vi "Set VLIM.vi"(8 "error in":errorcluster, 10 "VLIM":sgl, 11 "SR 3XX HVPS in":refnum<class "SR 3XX HVPS.lvclass">) -> (0 "error out":errorcluster, 3 "SR 3XX HVPS out":refnum<class "SR 3XX HVPS.lvclass">)   [LabVIEW 2014, in "SR 3XX HVPS.lvclass"]
doc: "The VLIM command sets the value of the voltage limit to x where x is the value in Volts. The sign of value x MUST match the PS300’s polarity setting.As with front panel control, the VLIM value must be greater than or equal to the VSET value or an execution error will be returned."
uses:
  SR 3XX HVPS.lvclass
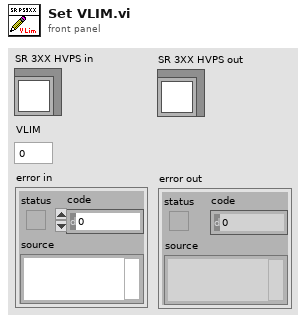
[diagram p1: front panel]
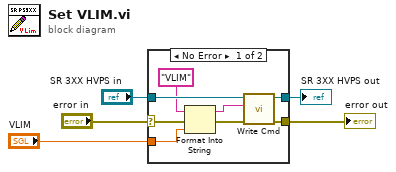
[diagram p0: block diagram]
diagram:
  n1 = case shown="No Error" "error in" {
    selector: "error in" -> [w7 w15]
    tunnel: [w11 w15] -> w4
    tunnel: [w12 w14] -> w2
    tunnel: "SR 3XX HVPS in" -> [w13 w14]
    tunnel: "VLIM" -> [w10 _]
    frame No Error {
      n2 = Format Into String(initial string="VLIM", error in=w7, w10) -> (resulting string=w8:string, error out=w6:errorcluster)  [unwired: 1 in]
      n3 = call "Write Cmd.vi"("error in"=w6, "Cmd"=w8, "SR 3XX HVPS in"=w13) -> ("error out"=w11:errorcluster, "SR 3XX HVPS out"=w12:refnum<class "SR 3XX HVPS.lvclass">)  [unwired: 7 in]
    }
    frame Error {
    }
  }
  "error out" <- w4
  "SR 3XX HVPS out" <- w2
